vi "数据表比对.vi"(6 "table输入 3":string(combo), 8 "error in (no error)":errorcluster, 9 "查询元素输入":string(combo), 10 "仪器日志参数":string, 11 "table输入":string(combo)) -> (0 "error out":errorcluster, 2 "待发送第一条数据":string[](array[string]), 3 "待发送数据":string[][](table), 4 "获取有效数据":string[][](array[string]))   [LabVIEW 2016]
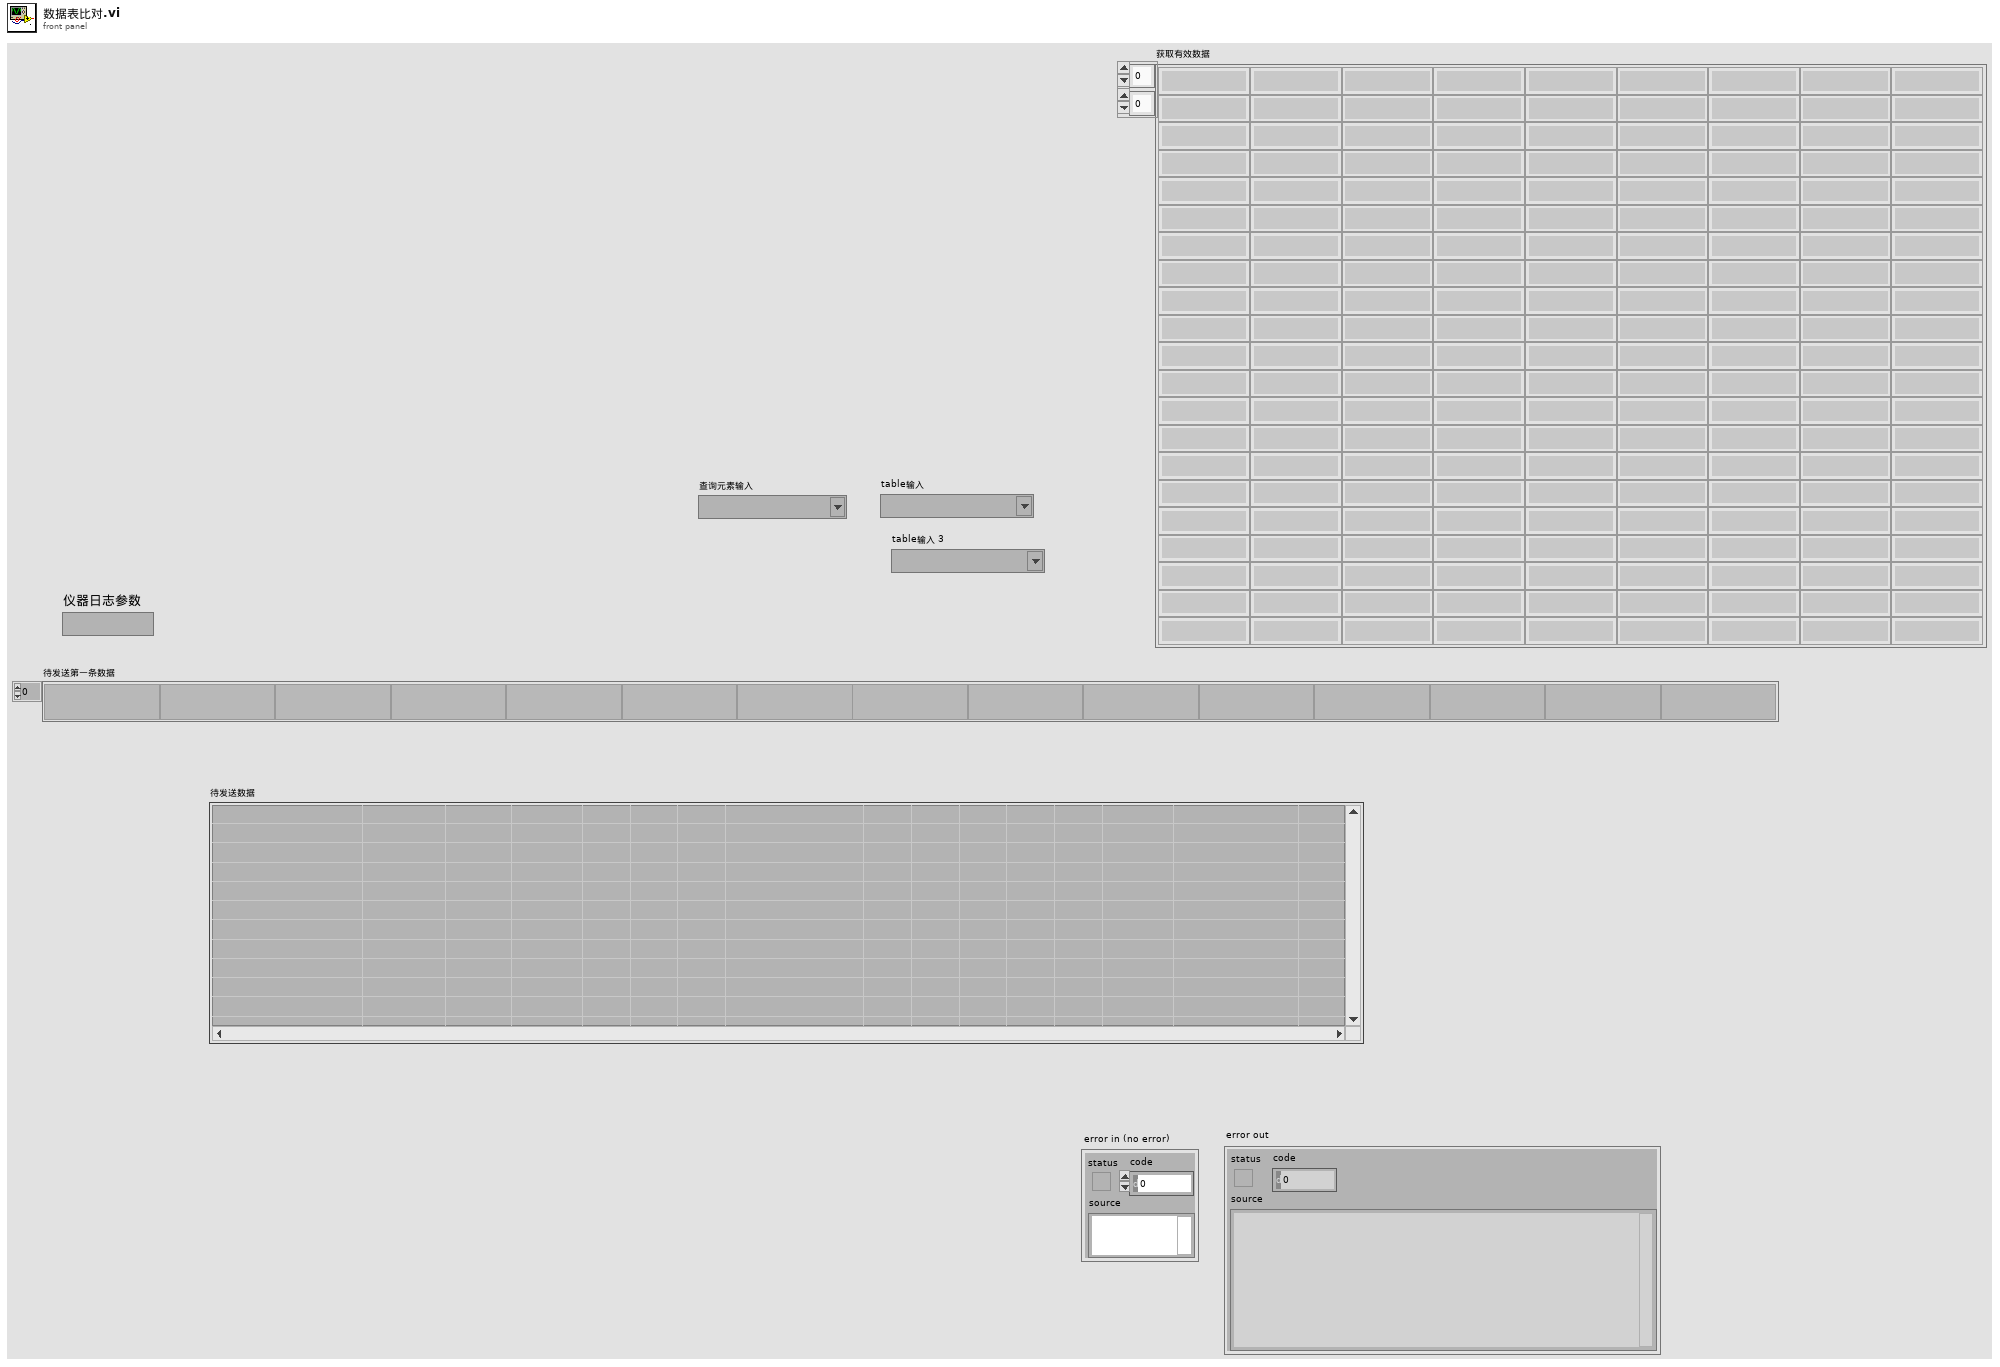
[diagram p1: front panel]
types:
  T1 = typedef "LVDateTimeRec.ctl" = cluster{"秒数的小数部分":dbl, "秒":i32, "分":i32, "时":i32, "日":i32, "月":i32, "年":i32, "天数（周）":i32, "天数（年）":i32, "DST":i32}
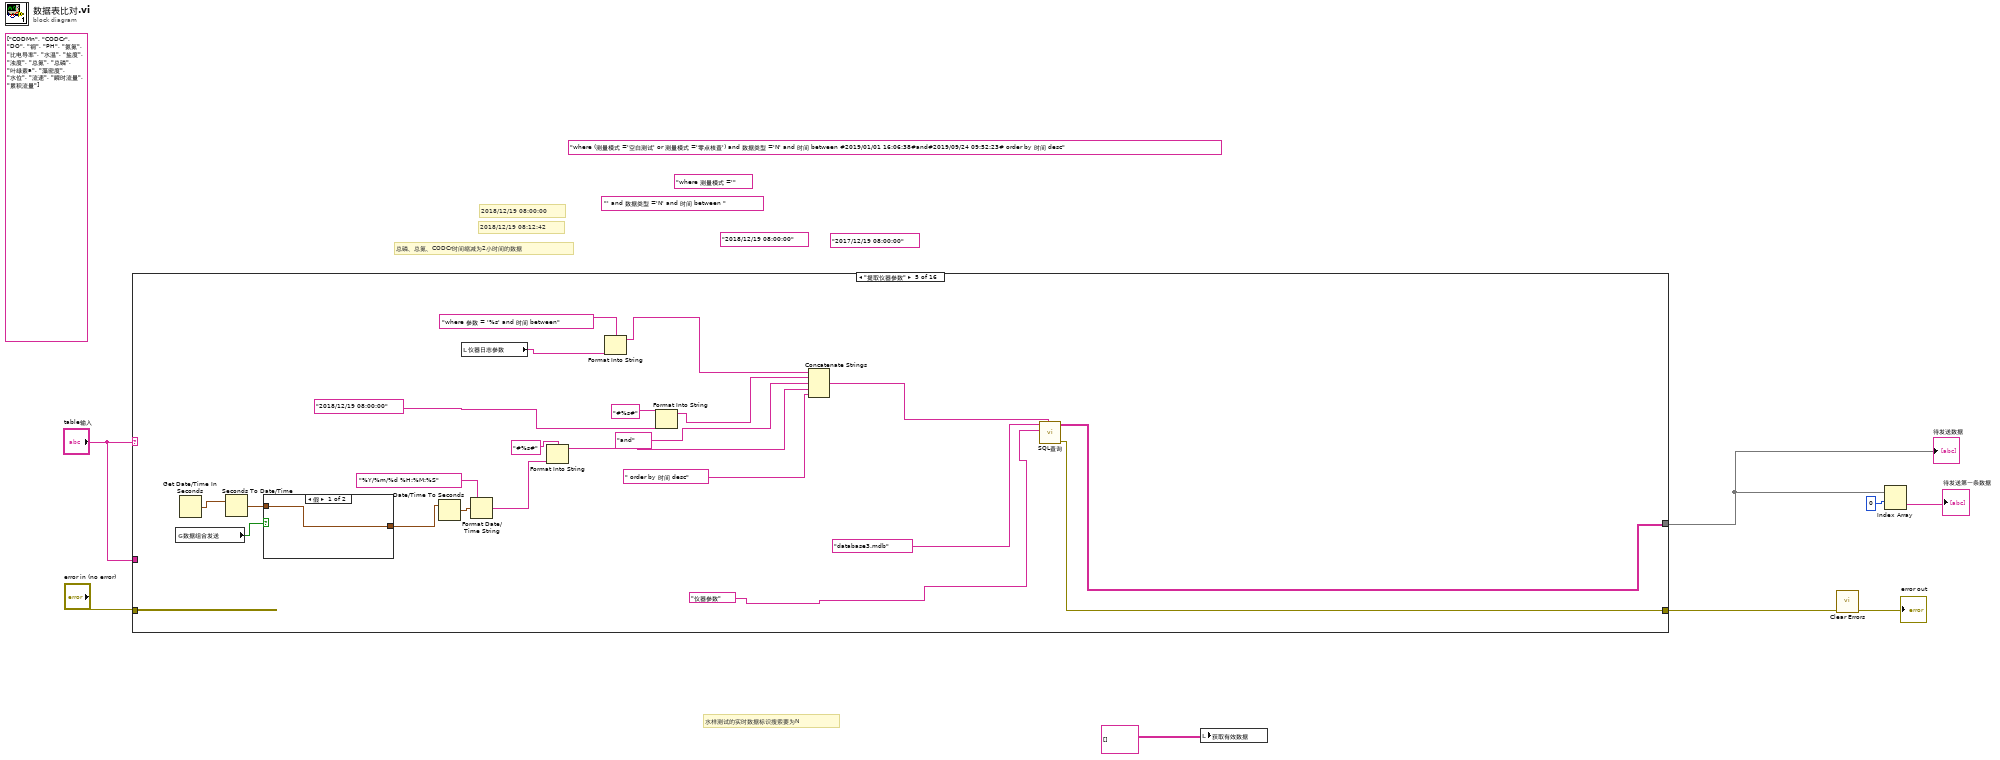
[diagram p0: block diagram]
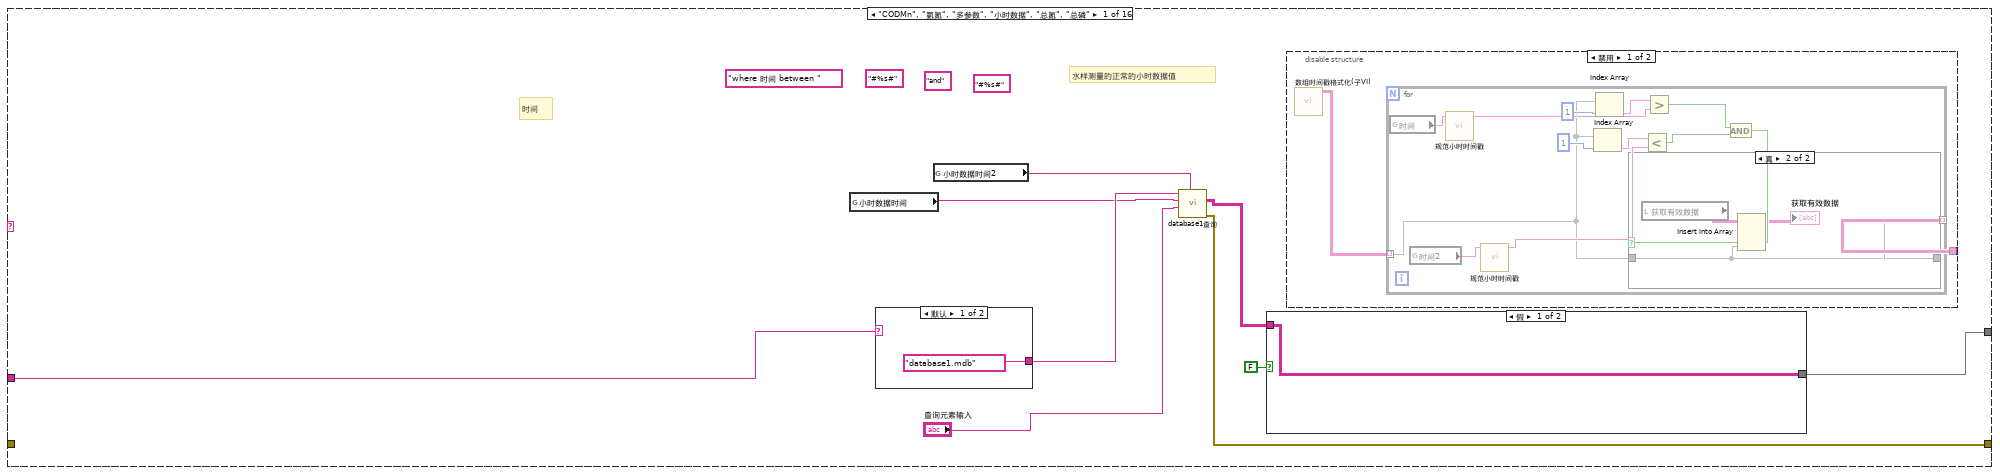
[diagram p2: hidden frame]
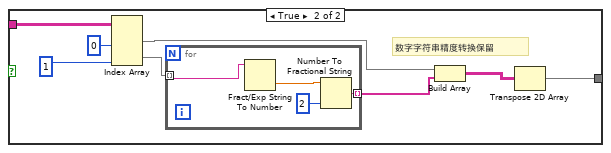
[diagram p3: hidden frame]
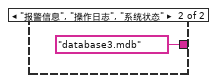
[diagram p6: hidden frame]
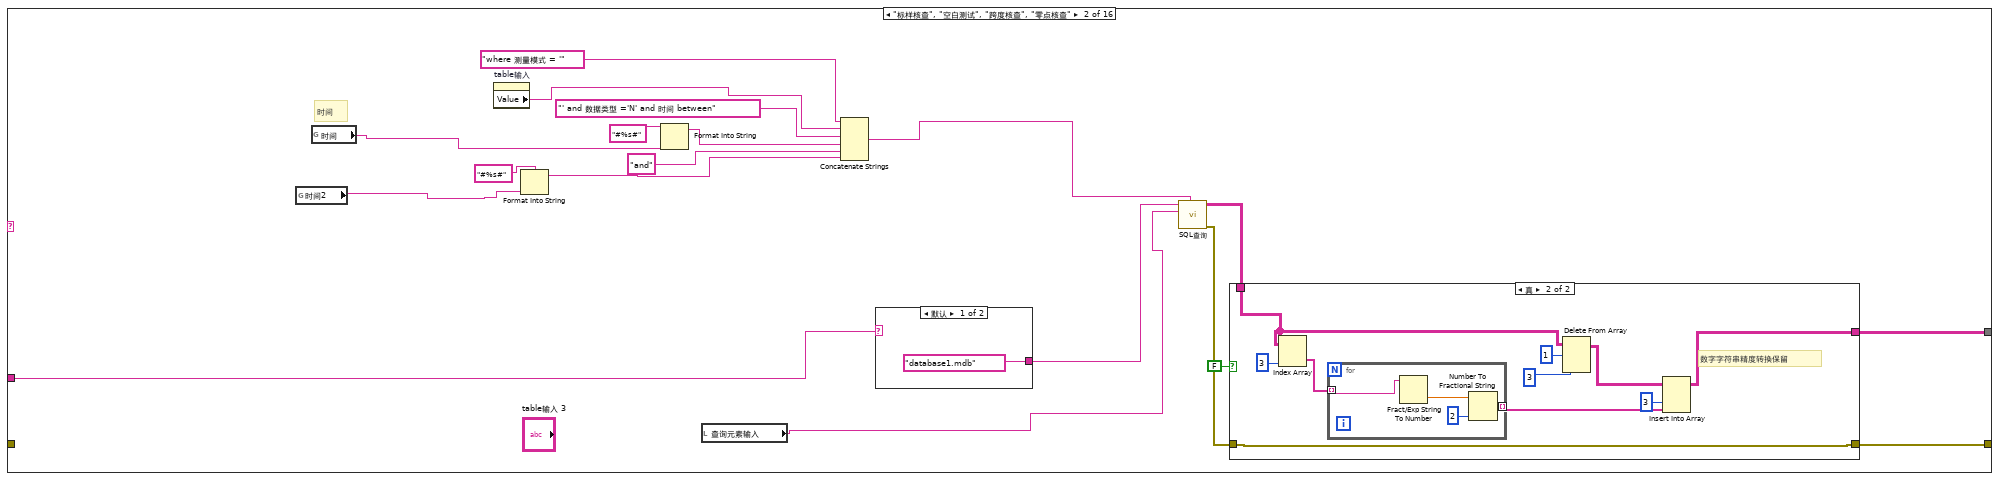
[diagram p7: hidden frame]
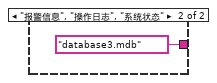
[diagram p9: hidden frame]
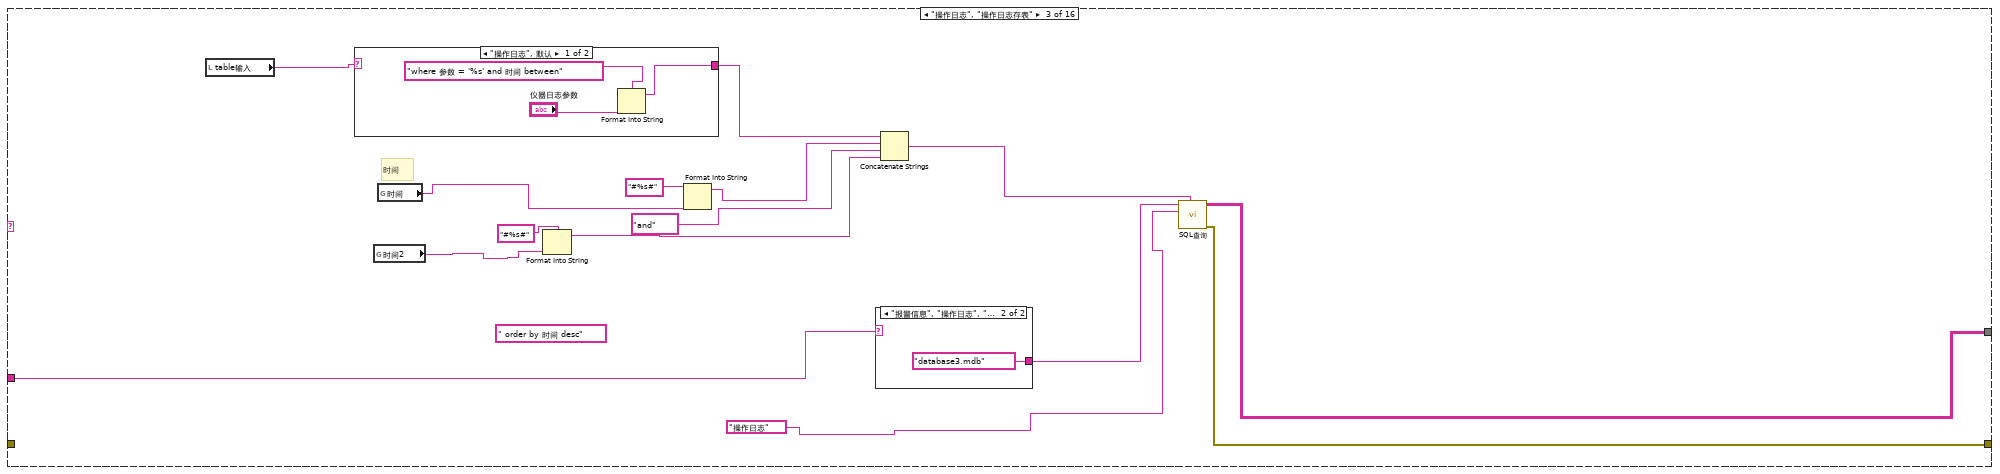
[diagram p10: hidden frame]
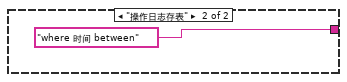
[diagram p11: hidden frame]
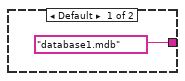
[diagram p12: hidden frame]
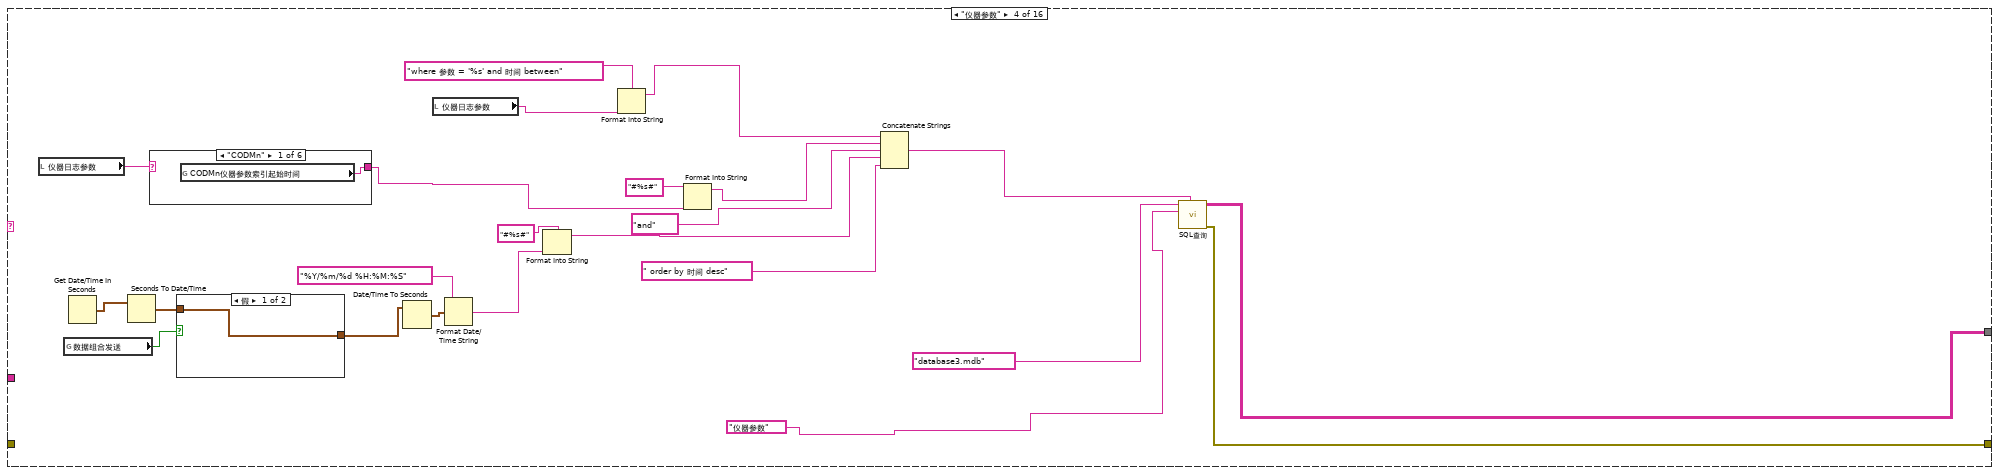
[diagram p13: hidden frame]
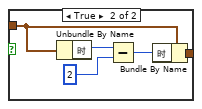
[diagram p14: hidden frame]
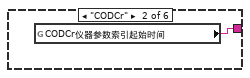
[diagram p15: hidden frame]
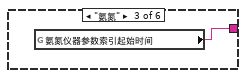
[diagram p16: hidden frame]
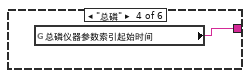
[diagram p17: hidden frame]
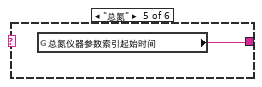
[diagram p18: hidden frame]
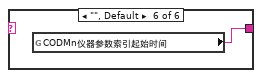
[diagram p19: hidden frame]
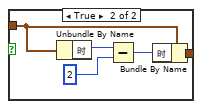
[diagram p20: hidden frame]
diagram:
  (unwired) "' and 数据类型 ='N' and 时间 between "
  (unwired) "where 测量模式 ='" ("condition")
  (unwired) "where (测量模式 ='空白测试' or 测量模式 ='零点核查') and 数据类型 ='N' and 时间 between #2019/01/01 16:06:38#and#2019/09/24 09:52:23# order by 时间 desc" ("condition")
  (unwired) string[] ["CODMn", "CODCr", "DO", "铜", "PH", "氨氮", "比电导率", "水温", "盐度", "浊度", "总氮", "总磷", "叶绿素a", "藻密度", "水位", "流速", "瞬时流量", "累积流量"] ("查询参数数组")
  (unwired) "2017/12/19 08:00:00"
  (unwired) "2018/12/19 08:00:00"
  # "水样测试的实时数据标识搜索要为N"
  # "2018/12/19 08:00:00"
  # "总磷、总氮、CODCr时间缩减为2小时间的数据"
  # "2018/12/19 08:12:42"
  n1 = case shown="\"提取仪器参数\"" "table输入" {
    tunnel: "error in (no error)" -> [_ _ _ _ _ _ _ w232 _ _ _ _ _ _ _ _]
    tunnel: [w14 w55 w100 w130 w164 w186 w219 w232 w247 w343 w390 w444 w499 w542 w585 w625] -> w6
    tunnel: [w10 w58 w98 w128 w162 w184 w217 w230 w250 w346 w393 w447 w502 w545 w588 w627] -> w1
    tunnel: "table输入" -> [w17 w69 w102 _ _ w174 w209 _ _ _ _ _ _ _ _ _]
    frame "CODMn", "氨氮", "多参数", "小时数据", "总氮", "总磷" {
      (unwired) "and" ("字符串")
      (unwired) "#%s#" ("初始字符串")
      (unwired) "#%s#" ("初始字符串")
      (unwired) "where 时间 between " ("condition")
      # "水样测量的正常的小时数据值"
      # "时间"
      n2 = global read "全局 水样时间.vi" "小时数据时间"() -> (w13:string)
      n3 = case shown="默认" w17 {
        tunnel: ["database1.mdb" ("database") "database3.mdb" ("database")] -> w16
        frame Default {
        }
        frame "报警信息", "操作日志", "系统状态" {
        }
      }
      n4 = global read "全局 时间2.vi" "小时数据时间2"() -> (w12:string)
      n5 = call "database1查询.vi"("时间2"=w12, "table"="查询元素输入", "时间1"=w13, "database"=w16) -> ("error out"=w14:errorcluster, "data"=w11:string[][])  [unwired: 4 in, 1 out]
      n6 = case shown="假" FALSE {
        tunnel: w11 -> [w18 w26]
        tunnel: [w18 w19] -> w10
        frame False {
        }
        frame True {
          # "数字字符串精度转换保留"
          n7 = Index Array(array=w26, index (col) #1=0 ("禁用的索引 (列)"), index (col) #2=1 ("索引 (列)")) -> (element #1=w22:string[], element #2=w23:string[])  [unwired: 2 in]
          n8 = for {
            tunnel: w23 -> [w28] mode=indexing
            tunnel: [w27] -> w21 mode=indexing
            n9 = Fract/Exp String To Number(string=w28) -> (number=w29:dbl)  [unwired: 3 in, 1 out]
            n10 = Number To Fractional String(number=w29, precision (6)=i16 2 ("精度(6)")) -> (F-format string=w27:string)  [unwired: 2 in]
          }
          n11 = Build Array(w22, w21) -> (w20:string[][])
          n12 = Transpose 2D Array(2D array=w20) -> (transposed array=w19:string[][])
        }
      }
      n13 = disable-structure shown="禁用" {
        disable-tunnel: [w31 _] -> _
        frame Disabled {
          n14 = call "数组时间戳格式化(子VI).vi"() -> ("待发送数据输出"=w32:string[][])  [unwired: 11 in]
          n15 = for {
            tunnel: w32 -> [w33] mode=indexing
            tunnel: [w35] -> w31 mode=indexing
            n16 = global read "全局 水样时间.vi" "时间"() -> (w39:string)
            n17 = global read "全局 时间2.vi" "时间2"() -> (w37:string)
            n18 = call "规范小时时间戳.vi"("字符串"=w39) -> ("result string"=w38:string)  [unwired: 10 in]
            n19 = call "规范小时时间戳.vi"("字符串"=w37) -> ("result string"=w36:string)  [unwired: 10 in]
            n20 = Index Array(array=w33, index=1 ("索引")) -> (element=w42:string)
            n21 = Index Array(array=w33, index=1 ("索引")) -> (element=w44:string)
            n22 = Less?(x=w42, y=w36) -> (x < y?=w41:bool)
            n23 = Greater?(x=w44, y=w38) -> (0:w40:bool)
            n24 = And(x=w40, y=w41) -> (x .and. y?=w34:bool)
            n25 = case shown="真" w34 {
              tunnel: w33 -> [_ w48]
              tunnel: [_ w48] -> w35
              frame False {
              }
              frame True {
                n26 = local read "获取有效数据"() -> (w47:string[][])
                n27 = Insert Into Array(array=w47, new element=w48) -> (→"获取有效数据":string[][])  [unwired: 2 in]
              }
            }
          }
        }
        frame Enabled {
        }
      }
    }
    frame "标样核查", "空白测试", "跨度核查", "零点核查" {
      # "时间"
      n28 = global read "全局 时间2.vi" "时间2"() -> (w60:string)
      n29 = global read "全局 水样时间.vi" "时间"() -> (w61:string)
      n30 = property on="table输入" class="CmbBox"() -> ("Value"=w51:string)  [unwired: 2 in, 2 out]
      n31 = Format Into String(format string="#%s#" ("初始字符串"), w60) -> (resulting string=w63:string)  [unwired: 2 in, 1 out]
      n32 = Format Into String(format string="#%s#" ("初始字符串"), w61) -> (resulting string=w67:string)  [unwired: 2 in, 1 out]
      n33 = local read "查询元素输入"() -> (w54:string)
      n34 = Concatenate Strings("where 测量模式 = '" ("condition"), w51, "' and 数据类型 ='N' and 时间 between" ("字符串"), w67, "and" ("字符串"), w63) -> (w62:string)
      n35 = case shown="默认" w69 {
        tunnel: ["database1.mdb" ("database") "database3.mdb" ("database")] -> w68
        frame Default {
        }
        frame "报警信息", "操作日志", "系统状态" {
        }
      }
      n36 = call "SQL查询.vi"("condition"=w62, "table输入"=w54, "database"=w68) -> ("error out"=w56:errorcluster, "data"=w59:string[][])  [unwired: 7 in]
      n37 = case shown="真" FALSE {
        tunnel: w59 -> [w71 w74]
        tunnel: [w71 w73] -> w58
        tunnel: [w70 w72] -> w55
        tunnel: w56 -> [w70 w72]
        frame False {
        }
        frame True {
          # "数字字符串精度转换保留"
          n38 = Index Array(array=w74, index (col)=3 ("禁用的索引 (列)")) -> (element=w80:string[])  [unwired: 1 in]
          n39 = for {
            tunnel: w80 -> [w83] mode=indexing
            tunnel: [w82] -> w76 mode=indexing
            n40 = Fract/Exp String To Number(string=w83) -> (number=w84:dbl)  [unwired: 3 in, 1 out]
            n41 = Number To Fractional String(number=w84, precision (6)=i16 2 ("精度(6)")) -> (F-format string=w82:string)  [unwired: 2 in]
          }
          n42 = Delete From Array(array=w74, length=1 ("长度"), index (col)=3 ("禁用的索引 (列)")) -> (array with subset deleted=w77:string[][])  [unwired: 1 in, 1 out]
          n43 = Insert Into Array(array=w77, index (col)=3 ("禁用的索引 (列)"), new element=w76) -> (w73:string[][])  [unwired: 1 in]
        }
      }
    }
    frame "操作日志", "操作日志存表" {
      (unwired) " order by 时间 desc" ("字符串")
      # "时间"
      n44 = local read "table输入"() -> (w90:string)
      n45 = case shown="\"操作日志\", 默认" w90 {
        tunnel: [w103 "where 时间 between" ("condition")] -> w89
        frame "操作日志", Default {
          n46 = Format Into String(format string="where 参数 = '%s' and 时间 between" ("condition"), "仪器日志参数") -> (resulting string=w103:string)  [unwired: 2 in, 1 out]
        }
        frame "操作日志存表" {
        }
      }
      n47 = global read "全局 时间2.vi" "时间2"() -> (w91:string)
      n48 = global read "全局 水样时间.vi" "时间"() -> (w92:string)
      n49 = Format Into String(format string="#%s#" ("初始字符串"), w91) -> (resulting string=w93:string)  [unwired: 2 in, 1 out]
      n50 = Format Into String(format string="#%s#" ("初始字符串"), w92) -> (resulting string=w97:string)  [unwired: 2 in, 1 out]
      n51 = case shown="\"报警信息\", \"操作日志\", \"操作日志存表\", \"系统状态\"" w102 {
        tunnel: ["database1.mdb" ("database") "database3.mdb" ("database")] -> w101
        frame Default {
        }
        frame "报警信息", "操作日志", "操作日志存表", "系统状态" {
        }
      }
      n52 = Concatenate Strings(w89, w97, "and" ("字符串"), w93) -> (w99:string)
      n53 = call "SQL查询.vi"("condition"=w99, "table输入"="操作日志", "database"=w101) -> ("error out"=w100:errorcluster, "data"=w98:string[][])  [unwired: 7 in]
    }
    frame "仪器参数" {
      n54 = local read "仪器日志参数"() -> (w109:string)
      n55 = global read "断电保存全局.vi" "数据组合发送"() -> (w116:bool)
      n56 = Get Date/Time In Seconds() -> (seconds since 1Jan1904=w111:timestamp)
      n57 = Seconds To Date/Time(time stamp (now)=w111) -> (date time rec=w114:T1)  [unwired: 1 in]
      n58 = case shown="\"CODMn\"" w109 {
        tunnel: [w138 w139 w140 w141 w142 w143] -> w117
        frame "CODMn" {
          n59 = global read "全局 时间2.vi" "CODMn仪器参数索引起始时间"() -> (w138:string)
        }
        frame "CODCr" {
          n60 = global read "全局 时间2.vi" "CODCr仪器参数索引起始时间"() -> (w139:string)
        }
        frame "氨氮" {
          n61 = global read "全局 时间2.vi" "氨氮仪器参数索引起始时间"() -> (w140:string)
        }
        frame "总磷" {
          n62 = global read "全局 时间2.vi" "总磷仪器参数索引起始时间"() -> (w141:string)
        }
        frame "总氮" {
          n63 = global read "全局 时间2.vi" "总氮仪器参数索引起始时间"() -> (w142:string)
        }
        frame "", Default {
          n64 = global read "全局 时间2.vi" "CODMn仪器参数索引起始时间"() -> (w143:string)
        }
      }
      n65 = case shown="假" w116 {
        tunnel: w114 -> [w132 w135]
        tunnel: [w132 w133] -> w115
        frame False {
        }
        frame True {
          n66 = Unbundle By Name(w135) -> ("时"=w137:i32)
          n67 = Subtract(x=w137, y=2) -> (x-y=w134:i32)
          n68 = Bundle By Name(cluster=w135, "时"=w134) -> (w133:T1)
        }
      }
      n69 = Date/Time To Seconds(2:w115) -> (0:w112:timestamp)  [unwired: 1 in]
      n70 = local read "仪器日志参数"() -> (w118:string)
      n71 = Format Date/Time String(time format string (%c)="%Y/%m/%d %H:%M:%S" ("时间格式字符串(%c)"), seconds (now)=w112) -> (date/time string=w110:string)  [unwired: 1 in]
      n72 = Format Into String(format string="#%s#" ("初始字符串"), w110) -> (resulting string=w123:string)  [unwired: 2 in, 1 out]
      n73 = Format Into String(format string="where 参数 = '%s' and 时间 between" ("condition"), w118) -> (resulting string=w122:string)  [unwired: 2 in, 1 out]
      n74 = Format Into String(format string="#%s#" ("初始字符串"), w117) -> (resulting string=w127:string)  [unwired: 2 in, 1 out]
      n75 = Concatenate Strings(w122, w127, "and" ("字符串"), w123, " order by 时间 desc" ("字符串")) -> (w129:string)
      n76 = call "SQL查询.vi"("condition"=w129, "table输入"="仪器参数", "database"="database3.mdb") -> ("error out"=w130:errorcluster, "data"=w128:string[][])  [unwired: 7 in]
    }
    frame "提取仪器参数" {
      n77 = global read "断电保存全局.vi" "数据组合发送"() -> (w151:bool)
      n78 = Get Date/Time In Seconds() -> (seconds since 1Jan1904=w146:timestamp)
      n79 = Seconds To Date/Time(time stamp (now)=w146) -> (date time rec=w149:T1)  [unwired: 1 in]
      n80 = case shown="假" w151 {
        tunnel: w149 -> [w166 w169]
        tunnel: [w166 w167] -> w150
        frame False {
        }
        frame True {
          n81 = Unbundle By Name(w169) -> ("时"=w171:i32)
          n82 = Subtract(x=w171, y=2) -> (x-y=w168:i32)
          n83 = Bundle By Name(cluster=w169, "时"=w168) -> (w167:T1)
        }
      }
      n84 = Date/Time To Seconds(2:w150) -> (0:w147:timestamp)  [unwired: 1 in]
      n85 = local read "仪器日志参数"() -> (w152:string)
      n86 = Format Date/Time String(time format string (%c)="%Y/%m/%d %H:%M:%S" ("时间格式字符串(%c)"), seconds (now)=w147) -> (date/time string=w145:string)  [unwired: 1 in]
      n87 = Format Into String(format string="#%s#" ("初始字符串"), w145) -> (resulting string=w157:string)  [unwired: 2 in, 1 out]
      n88 = Format Into String(format string="where 参数 = '%s' and 时间 between" ("condition"), w152) -> (resulting string=w156:string)  [unwired: 2 in, 1 out]
      n89 = Format Into String(format string="#%s#" ("初始字符串"), "2018/12/19 08:00:00") -> (resulting string=w161:string)  [unwired: 2 in, 1 out]
      n90 = Concatenate Strings(w156, w161, "and" ("字符串"), w157, " order by 时间 desc" ("字符串")) -> (w163:string)
      n91 = call "SQL查询.vi"("condition"=w163, "table输入"="仪器参数", "database"="database3.mdb") -> ("error out"=w164:errorcluster, "data"=w162:string[][])  [unwired: 7 in]
    }
    frame "报警信息", "报警信息存表" {
      # "时间"
      n92 = local read "table输入"() -> (w173:string)
      n93 = case shown="\"环境参数\"" w173 {
        tunnel: [w193 w196 "where 时间 between" ("condition")] -> w176
        frame "报警信息", Default {
          n94 = local read "仪器日志参数"() -> (w192:string)
          n95 = Format Into String(format string="where 参数 = '%s' and 时间 between" ("condition"), w192) -> (resulting string=w193:string)  [unwired: 2 in, 1 out]
        }
        frame "环境参数" {
          n96 = local read "仪器日志参数"() -> (w195:string)
          n97 = Format Into String(format string="where 参数 = '%s' and 时间 between" ("condition"), w195) -> (resulting string=w196:string)  [unwired: 2 in, 1 out]
        }
        frame "报警信息存表" {
        }
      }
      n98 = global read "全局 时间2.vi" "时间2"() -> (w177:string)
      n99 = global read "全局 水样时间.vi" "时间"() -> (w178:string)
      n100 = case shown="\"环境参数\"" w173 {
        tunnel: [" order by 时间 desc" ("字符串") "" ("仪器日志参数")] -> w172
        frame "环境参数" {
        }
        frame "报警信息", Default {
        }
      }
      n101 = Format Into String(format string="#%s#" ("初始字符串"), w177) -> (resulting string=w179:string)  [unwired: 2 in, 1 out]
      n102 = case shown="\"报警信息\", 默认" w174 {
        tunnel: [w190 "报警信息" ("table输入")] -> w175
        frame "环境参数" {
          n103 = local read "仪器日志参数"() -> (w190:string)
        }
        frame "报警信息", Default {
        }
      }
      n104 = Format Into String(format string="#%s#" ("初始字符串"), w178) -> (resulting string=w183:string)  [unwired: 2 in, 1 out]
      n105 = case shown="默认" w174 {
        tunnel: ["database1.mdb" ("database") "database3.mdb" ("database")] -> w187
        frame Default {
        }
        frame "报警信息", "报警信息存表", "操作日志", "系统状态" {
        }
      }
      n106 = Concatenate Strings(w176, w183, "and" ("字符串"), w179, w172) -> (w185:string)
      n107 = call "SQL查询.vi"("condition"=w185, "table输入"=w175, "database"=w187) -> ("error out"=w186:errorcluster, "data"=w184:string[][])  [unwired: 7 in]
    }
    frame "环境参数" {
      n108 = local read "table输入"() -> (w208:string)
      n109 = Get Date/Time In Seconds() -> (seconds since 1Jan1904=w205:timestamp)
      n110 = Seconds To Date/Time(time stamp (now)=w205) -> (date time rec=w202:T1)  [unwired: 1 in]
      n111 = case shown="\"环境参数\"" w208 {
        tunnel: [w224 "where 时间 between" ("condition") "where 时间 between" ("condition")] -> w211
        frame "报警信息", Default {
          n112 = local read "仪器日志参数"() -> (w223:string)
          n113 = Format Into String(format string="where 参数 = '%s' and 时间 between" ("condition"), w223) -> (resulting string=w224:string)  [unwired: 2 in, 1 out]
        }
        frame "环境参数" {
        }
        frame "报警信息存表" {
        }
      }
      n114 = Date/Time To Seconds(2:w202) -> (0:w204:timestamp)  [unwired: 1 in]
      n115 = Format Date/Time String(time format string (%c)="%Y/%m/%d %H:%M:%S" ("时间格式字符串(%c)"), seconds (now)=w204) -> (date/time string=w201:string)  [unwired: 1 in]
      n116 = Format Into String(format string="#%s#" ("初始字符串"), w201) -> (resulting string=w212:string)  [unwired: 2 in, 1 out]
      n117 = case shown="\"环境参数\"" w209 {
        tunnel: [w221 "报警信息" ("table输入")] -> w210
        frame "环境参数" {
          n118 = local read "仪器日志参数"() -> (w221:string)
        }
        frame "报警信息", Default {
        }
      }
      n119 = Format Into String(format string="#%s#" ("初始字符串"), "1904/01/01 00:00:00") -> (resulting string=w216:string)  [unwired: 2 in, 1 out]
      n120 = case shown="默认" w209 {
        tunnel: ["database1.mdb" ("database") "database3.mdb" ("database")] -> w220
        frame Default {
        }
        frame "报警信息", "报警信息存表", "操作日志", "系统状态" {
        }
      }
      n121 = Concatenate Strings(w211, w216, "and" ("字符串"), w212, " order by 时间 desc" ("字符串")) -> (w218:string)
      n122 = call "SQL查询.vi"("condition"=w218, "table输入"=w210, "database"=w220) -> ("error out"=w219:errorcluster, "data"=w217:string[][])  [unwired: 7 in]
    }
    frame Default {
      # "时间格式转换"
      n123 = local read "待发送数据"() -> (w231:string[][])
      n124 = call "数组时间戳格式化(子VI).vi"("待发送数据输入"=w231) -> ("待发送数据输出"=w230:string[][])  [unwired: 10 in]
    }
    frame "实时数据" {
      # "空白测试or零点核查要加括号"
      # "上传本地时间点的实时数据"
      # "上传质控数据（空白测试，跨度核查，核查数据，平行样数据）"
      n125 = global read "全局 实时数据参数.vi" "实时数据参数"() -> (w242:string)
      n126 = global read "断电保存全局.vi" "数据组合发送"() -> (w234:bool)
      n127 = Get Date/Time In Seconds() -> (seconds since 1Jan1904=w241:timestamp)
      n128 = case shown="\"空白测试\"" w242 {
        tunnel: [w267 w289 w300 w306] -> w243
        tunnel: w242 -> [w263 w287 _ w302]
        tunnel: [w266 w283 w296 w301] -> w237
        frame "水样测试" {
          n129 = Get Date/Time In Seconds() -> (seconds since 1Jan1904=w275:timestamp)
          n130 = local read "查询元素输入"() -> (w268:string)
          n131 = Format Date/Time String(time format string (%c)="%Y%m%d%H%M%S%3u" ("时间格式字符串(%c)"), seconds (now)=w275) -> (date/time string=w273:string)  [unwired: 1 in]
          n132 = Replace Substring(2:8 ("长度（子字符串长度）"), 3:10 ("偏移量(0)"), 4:"0000" ("子字符串(\"\")"), 5:w273) -> (1:w269:string)  [unwired: 1 out]
          n133 = case shown="默认" w268 {
            tunnel: w269 -> [w277 w280 _]
            tunnel: [w276 w281 w282] -> w267
            frame Default {
              n134 = Search and Replace String(input string=w277, search string="." ("搜索字符串")) -> (result string=w278:string)  [unwired: 6 in, 3 out]
              n135 = call "格式时间字符串.vi"("字符串"=w278) -> ("连接的字符串"=w276:string)  [unwired: 10 in]
            }
            frame "CODCr", "CODMn", "累积流量", "总氮", "总磷" {
              n136 = call "实时数据查询用2小时间的数据.vi"("字符串"=w280) -> ("连接的字符串"=w281:string)  [unwired: 10 in]
            }
            frame "CODCr加标回收率", "CODMn加标回收率", "氨氮加标回收率", "总氮加标回收率", "总磷加标回收率" {
              n137 = global read "全局 时间2.vi" "加标回收索引起始时间"() -> (w282:string)
            }
          }
          n138 = Concatenate Strings("where 测量模式 ='" ("condition"), w263, "' and 数据类型 ='N' and 时间 between ") -> (w266:string)
        }
        frame "空白测试" {
          n139 = local read "查询元素输入"() -> (w288:string)
          n140 = case shown="\"氨氮\"" w288 {
            tunnel: [w290 w291 w292 w293 w294 w295] -> w289
            frame "CODMn" {
              n141 = global read "全局 时间2.vi" "CODMn零点核查索引起始时间"() -> (w290:string)
            }
            frame "CODCr" {
              n142 = global read "全局 时间2.vi" "CODCr零点核查索引起始时间"() -> (w291:string)
            }
            frame "氨氮" {
              n143 = global read "全局 时间2.vi" "氨氮零点核查索引起始时间"() -> (w292:string)
            }
            frame "总磷" {
              n144 = global read "全局 时间2.vi" "总磷零点核查索引起始时间"() -> (w293:string)
            }
            frame "总氮" {
              n145 = global read "全局 时间2.vi" "总氮零点核查索引起始时间"() -> (w294:string)
            }
            frame "", Default {
              n146 = global read "全局 时间2.vi" "零点核查索引起始时间"() -> (w295:string)
            }
          }
          n147 = Concatenate Strings("where (测量模式 ='" ("condition"), w287, "' or 测量模式 = '零点核查", "') and 数据类型 ='N' and 时间 between ") -> (w283:string)
        }
        frame "核查数据" {
          n148 = global read "全局 时间2.vi" "标样核查索引起始时间"() -> (w300:string)
          n149 = Concatenate Strings("where 测量模式 ='" ("condition"), "标样核查" ("实时数据参数"), "' and 数据类型 ='N' and 时间 between ") -> (w296:string)
        }
        frame "跨度核查", Default {
          n150 = local read "查询元素输入"() -> (w305:string)
          n151 = case shown="\"氨氮\"" w305 {
            tunnel: [w307 w308 w309 w310 w311 w312] -> w306
            frame "CODMn" {
              n152 = global read "全局 时间2.vi" "CODMn跨度核查索引起始时间"() -> (w307:string)
            }
            frame "CODCr" {
              n153 = global read "全局 时间2.vi" "CODCr跨度核查索引起始时间"() -> (w308:string)
            }
            frame "氨氮" {
              n154 = global read "全局 时间2.vi" "氨氮跨度核查索引起始时间"() -> (w309:string)
            }
            frame "总磷" {
              n155 = global read "全局 时间2.vi" "总磷跨度核查索引起始时间"() -> (w310:string)
            }
            frame "总氮" {
              n156 = global read "全局 时间2.vi" "总氮跨度核查索引起始时间"() -> (w311:string)
            }
            frame "", Default {
              n157 = global read "全局 时间2.vi" "跨度核查索引起始时间"() -> (w312:string)
            }
          }
          n158 = Concatenate Strings("where 测量模式 ='" ("condition"), w302, "' and 数据类型 ='N' and 时间 between ") -> (w301:string)
        }
      }
      n159 = Seconds To Date/Time(time stamp (now)=w241) -> (date time rec=w236:T1)  [unwired: 1 in]
      n160 = case shown="假" w234 {
        tunnel: w236 -> [w257 w260]
        tunnel: [w257 w258] -> w235
        frame False {
        }
        frame True {
          n161 = Unbundle By Name(w260) -> ("时"=w262:i32)
          n162 = Subtract(x=w262, y=2) -> (x-y=w259:i32)
          n163 = Bundle By Name(cluster=w260, "时"=w259) -> (w258:T1)
        }
      }
      n164 = Date/Time To Seconds(2:w235) -> (0:w240:timestamp)  [unwired: 1 in]
      n165 = Format Date/Time String(time format string (%c)="%Y/%m/%d %H:%M:%S" ("时间格式字符串(%c)"), seconds (now)=w240) -> (date/time string=w238:string)  [unwired: 1 in]
      n166 = local read "查询元素输入"() -> (w246:string)
      n167 = Format Into String(format string="#%s#" ("初始字符串"), w238) -> (resulting string=w252:string)  [unwired: 2 in, 1 out]
      n168 = Format Into String(format string="#%s#" ("初始字符串"), w243) -> (resulting string=w256:string)  [unwired: 2 in, 1 out]
      n169 = Concatenate Strings(w237, w256, "and" ("字符串"), w252, " order by 时间 desc" ("字符串")) -> (w245:string)
      n170 = call "SQL查询.vi"("condition"=w245, "table输入"=w246, "database"="database1.mdb") -> ("error out"=w248:errorcluster, "data"=w244:string[][])  [unwired: 7 in]
      n171 = case shown="假" FALSE {
        tunnel: [w317 w320] -> w250
        tunnel: w244 -> [w317 w319]
        tunnel: w248 -> [w316 w318]
        tunnel: [w316 w318] -> w247
        frame False {
        }
        frame True {
          # "数字字符串精度转换保留"
          n172 = Index Array(array=w319, index (col)=3 ("禁用的索引 (列)")) -> (element=w326:string[])  [unwired: 1 in]
          n173 = for {
            tunnel: w326 -> [w329] mode=indexing
            tunnel: [w328] -> w322 mode=indexing
            n174 = Fract/Exp String To Number(string=w329) -> (number=w330:dbl)  [unwired: 3 in, 1 out]
            n175 = Number To Fractional String(number=w330, precision (6)=i16 2 ("精度(6)")) -> (F-format string=w328:string)  [unwired: 2 in]
          }
          n176 = Delete From Array(array=w319, length=1 ("长度"), index (col)=3 ("禁用的索引 (列)")) -> (array with subset deleted=w323:string[][])  [unwired: 1 in, 1 out]
          n177 = Insert Into Array(array=w323, index (col)=3 ("禁用的索引 (列)"), new element=w322) -> (w320:string[][])  [unwired: 1 in]
        }
      }
      n178 = case shown="默认" w246 {
        tunnel: w246 -> [_ w315]
        tunnel: w245 -> [_ w314]
        tunnel: w244 -> [_ w313]
        frame Default {
        }
        frame "CODCr", "总氮", "总磷" {
          n179 = global write "全局 实时数据参数.vi" "参数"(w315) -> ()
          n180 = global write "全局 实时数据参数.vi" "连接的字符串"(w314) -> ()
          n181 = global write "全局 实时数据参数.vi" "data"(w313) -> ()
        }
      }
    }
    frame "加标回收" {
      w338 = "加标回收率" ("字符串")
      # "上传本地时间点的实时数据"
      # "上传加标回收数据"
      n182 = global read "全局 数据发送重叠.vi" "掉线指示灯"() -> (w339:bool)
      n183 = case shown="假" w339 {
        tunnel: [w355 w359] -> w340
        frame False {
          n184 = global read "全局 数据发送重叠.vi" "数据发送重叠"() -> (w356:bool)
          n185 = case shown="假" w356 {
            tunnel: [w357 w358] -> w355
            frame False {
              n186 = global read "全局 时间2.vi" "加标回收索引起始时间"() -> (w357:string)
            }
            frame True {
              n187 = global read "全局 数据发送重叠.vi" "数据发送重叠开始时间戳"() -> (w358:string)
            }
          }
        }
        frame True {
          n188 = global read "全局 数据发送重叠.vi" "TCP掉线时间节点"() -> (w359:string)
        }
      }
      n189 = Get Date/Time In Seconds() -> (seconds since 1Jan1904=w336:timestamp)
      n190 = Seconds To Date/Time(time stamp (now)=w336) -> (date time rec=w333:T1)  [unwired: 1 in]
      n191 = Date/Time To Seconds(2:w333) -> (0:w335:timestamp)  [unwired: 1 in]
      n192 = Format Date/Time String(time format string (%c)="%Y/%m/%d %H:%M:%S" ("时间格式字符串(%c)"), seconds (now)=w335) -> (date/time string=w332:string)  [unwired: 1 in]
      n193 = local read "查询元素输入"() -> (w337:string)
      n194 = Format Into String(format string="#%s#" ("初始字符串"), w332) -> (resulting string=w350:string)  [unwired: 2 in, 1 out]
      n195 = Format Into String(format string="#%s#" ("初始字符串"), w340) -> (resulting string=w354:string)  [unwired: 2 in, 1 out]
      n196 = Concatenate Strings("where 参数 ='" ("condition"), w337, "' and 时间 between ", w354, "and" ("字符串"), w350) -> (w342:string)
      n197 = call "SQL查询.vi"("condition"=w342, "table输入"=w338, "database"="database1.mdb") -> ("error out"=w344:errorcluster, "data"=w341:string[][])  [unwired: 7 in]
      n198 = case shown="假" FALSE {
        tunnel: [w364 w367] -> w346
        tunnel: w341 -> [w364 w366]
        tunnel: w344 -> [w363 w365]
        tunnel: [w363 w365] -> w343
        frame False {
        }
        frame True {
          # "数字字符串精度转换保留"
          n199 = Index Array(array=w366, index (col)=3 ("禁用的索引 (列)")) -> (element=w373:string[])  [unwired: 1 in]
          n200 = for {
            tunnel: w373 -> [w376] mode=indexing
            tunnel: [w375] -> w369 mode=indexing
            n201 = Fract/Exp String To Number(string=w376) -> (number=w377:dbl)  [unwired: 3 in, 1 out]
            n202 = Number To Fractional String(number=w377, precision (6)=i16 2 ("精度(6)")) -> (F-format string=w375:string)  [unwired: 2 in]
          }
          n203 = Delete From Array(array=w366, length=1 ("长度"), index (col)=3 ("禁用的索引 (列)")) -> (array with subset deleted=w370:string[][])  [unwired: 1 in, 1 out]
          n204 = Insert Into Array(array=w370, index (col)=3 ("禁用的索引 (列)"), new element=w369) -> (w367:string[][])  [unwired: 1 in]
        }
      }
      n205 = case shown="\"CODCr\", \"总氮\", \"总磷\"" w338 {
        tunnel: w338 -> [_ w362]
        tunnel: w342 -> [_ w361]
        tunnel: w341 -> [_ w360]
        frame Default {
        }
        frame "CODCr", "总氮", "总磷" {
          n206 = global write "全局 实时数据参数.vi" "参数"(w362) -> ()
          n207 = global write "全局 实时数据参数.vi" "连接的字符串"(w361) -> ()
          n208 = global write "全局 实时数据参数.vi" "data"(w360) -> ()
        }
      }
    }
    frame "平行样测试" {
      w385 = "平行样测试" ("字符串")
      # "上传本地时间点的实时数据"
      # "上传平行样数据"
      n209 = global read "全局 数据发送重叠.vi" "掉线指示灯"() -> (w386:bool)
      n210 = case shown="假" w386 {
        tunnel: [w402 w413] -> w387
        frame False {
          n211 = global read "全局 数据发送重叠.vi" "数据发送重叠"() -> (w403:bool)
          n212 = case shown="假" w403 {
            tunnel: [w404 w412] -> w402
            frame False {
              n213 = local read "查询元素输入"() -> (w405:string)
              n214 = case shown="\"CODCr\"" w405 {
                tunnel: [w406 w407 w408 w409 w410 w411] -> w404
                frame "CODMn" {
                  n215 = global read "全局 时间2.vi" "CODMn平行样索引起始时间"() -> (w406:string)
                }
                frame "CODCr" {
                  n216 = global read "全局 时间2.vi" "CODCr平行样索引起始时间"() -> (w407:string)
                }
                frame "氨氮" {
                  n217 = global read "全局 时间2.vi" "氨氮平行样索引起始时间"() -> (w408:string)
                }
                frame "总磷" {
                  n218 = global read "全局 时间2.vi" "总磷平行样索引起始时间"() -> (w409:string)
                }
                frame "总氮" {
                  n219 = global read "全局 时间2.vi" "总磷平行样索引起始时间"() -> (w410:string)
                }
                frame "", Default {
                  n220 = global read "全局 时间2.vi" "平行样索引起始时间"() -> (w411:string)
                }
              }
            }
            frame True {
              n221 = global read "全局 数据发送重叠.vi" "数据发送重叠开始时间戳"() -> (w412:string)
            }
          }
        }
        frame True {
          n222 = global read "全局 数据发送重叠.vi" "TCP掉线时间节点"() -> (w413:string)
        }
      }
      n223 = Get Date/Time In Seconds() -> (seconds since 1Jan1904=w383:timestamp)
      n224 = Seconds To Date/Time(time stamp (now)=w383) -> (date time rec=w380:T1)  [unwired: 1 in]
      n225 = Date/Time To Seconds(2:w380) -> (0:w382:timestamp)  [unwired: 1 in]
      n226 = Format Date/Time String(time format string (%c)="%Y/%m/%d %H:%M:%S" ("时间格式字符串(%c)"), seconds (now)=w382) -> (date/time string=w379:string)  [unwired: 1 in]
      n227 = local read "查询元素输入"() -> (w384:string)
      n228 = Format Into String(format string="#%s#" ("初始字符串"), w379) -> (resulting string=w397:string)  [unwired: 2 in, 1 out]
      n229 = Format Into String(format string="#%s#" ("初始字符串"), w387) -> (resulting string=w401:string)  [unwired: 2 in, 1 out]
      n230 = Concatenate Strings("where 参数 ='" ("condition"), w384, "' and 时间 between ", w401, "and" ("字符串"), w397) -> (w389:string)
      n231 = call "SQL查询.vi"("condition"=w389, "table输入"=w385, "database"="database1.mdb") -> ("error out"=w391:errorcluster, "data"=w388:string[][])  [unwired: 7 in]
      n232 = case shown="假" FALSE {
        tunnel: [w418 w421] -> w393
        tunnel: w388 -> [w418 w420]
        tunnel: w391 -> [w417 w419]
        tunnel: [w417 w419] -> w390
        frame False {
        }
        frame True {
          # "数字字符串精度转换保留"
          n233 = Index Array(array=w420, index (col)=3 ("禁用的索引 (列)")) -> (element=w427:string[])  [unwired: 1 in]
          n234 = for {
            tunnel: w427 -> [w430] mode=indexing
            tunnel: [w429] -> w423 mode=indexing
            n235 = Fract/Exp String To Number(string=w430) -> (number=w431:dbl)  [unwired: 3 in, 1 out]
            n236 = Number To Fractional String(number=w431, precision (6)=i16 2 ("精度(6)")) -> (F-format string=w429:string)  [unwired: 2 in]
          }
          n237 = Delete From Array(array=w420, length=1 ("长度"), index (col)=3 ("禁用的索引 (列)")) -> (array with subset deleted=w424:string[][])  [unwired: 1 in, 1 out]
          n238 = Insert Into Array(array=w424, index (col)=3 ("禁用的索引 (列)"), new element=w423) -> (w421:string[][])  [unwired: 1 in]
        }
      }
      n239 = case shown="默认" w385 {
        tunnel: w385 -> [_ w416]
        tunnel: w389 -> [_ w415]
        tunnel: w388 -> [_ w414]
        frame Default {
        }
        frame "CODCr", "总氮", "总磷" {
          n240 = global write "全局 实时数据参数.vi" "参数"(w416) -> ()
          n241 = global write "全局 实时数据参数.vi" "连接的字符串"(w415) -> ()
          n242 = global write "全局 实时数据参数.vi" "data"(w414) -> ()
        }
      }
    }
    frame "集成干预测试" {
      w439 = "集成干预测试" ("字符串")
      # "上传本地时间点的实时数据"
      # "上传集成干预数据"
      n243 = global read "全局 数据发送重叠.vi" "掉线指示灯"() -> (w440:bool)
      n244 = case shown="假" w440 {
        tunnel: [w456 w472] -> w441
        frame False {
          n245 = global read "全局 数据发送重叠.vi" "数据发送重叠"() -> (w457:bool)
          n246 = case shown="假" w457 {
            tunnel: [w458 w471] -> w456
            frame False {
              n247 = local read "查询元素输入"() -> (w459:string)
              n248 = case shown="\"浊度\"" w459 {
                tunnel: [w460 w461 w462 w463 w464 w465 w466 w467 w468 w469 w470] -> w458
                frame "CODMn" {
                  n249 = global read "全局 时间2.vi" "CODMn集成干预索引起始时间"() -> (w460:string)
                }
                frame "CODCr" {
                  n250 = global read "全局 时间2.vi" "CODCr集成干预索引起始时间"() -> (w461:string)
                }
                frame "氨氮" {
                  n251 = global read "全局 时间2.vi" "氨氮集成干预索引起始时间"() -> (w462:string)
                }
                frame "总磷" {
                  n252 = global read "全局 时间2.vi" "总磷集成干预索引起始时间"() -> (w463:string)
                }
                frame "总氮" {
                  n253 = global read "全局 时间2.vi" "总氮集成干预索引起始时间"() -> (w464:string)
                }
                frame "DO" {
                  n254 = global read "全局 时间2.vi" "DO集成干预索引起始时间"() -> (w465:string)
                }
                frame "PH" {
                  n255 = global read "全局 时间2.vi" "PH集成干预索引起始时间"() -> (w466:string)
                }
                frame "比电导率" {
                  n256 = global read "全局 时间2.vi" "比电导率集成干预索引起始时间"() -> (w467:string)
                }
                frame "水温" {
                  n257 = global read "全局 时间2.vi" "水温集成干预索引起始时间"() -> (w468:string)
                }
                frame "浊度" {
                  n258 = global read "全局 时间2.vi" "浊度集成干预索引起始时间"() -> (w469:string)
                }
                frame "", Default {
                  n259 = global read "全局 时间2.vi" "平行样索引起始时间"() -> (w470:string)
                }
              }
            }
            frame True {
              n260 = global read "全局 数据发送重叠.vi" "数据发送重叠开始时间戳"() -> (w471:string)
            }
          }
        }
        frame True {
          n261 = global read "全局 数据发送重叠.vi" "TCP掉线时间节点"() -> (w472:string)
        }
      }
      n262 = Get Date/Time In Seconds() -> (seconds since 1Jan1904=w437:timestamp)
      n263 = Seconds To Date/Time(time stamp (now)=w437) -> (date time rec=w434:T1)  [unwired: 1 in]
      n264 = Date/Time To Seconds(2:w434) -> (0:w436:timestamp)  [unwired: 1 in]
      n265 = Format Date/Time String(time format string (%c)="%Y/%m/%d %H:%M:%S" ("时间格式字符串(%c)"), seconds (now)=w436) -> (date/time string=w433:string)  [unwired: 1 in]
      n266 = local read "查询元素输入"() -> (w438:string)
      n267 = Format Into String(format string="#%s#" ("初始字符串"), w433) -> (resulting string=w451:string)  [unwired: 2 in, 1 out]
      n268 = Format Into String(format string="#%s#" ("初始字符串"), w441) -> (resulting string=w455:string)  [unwired: 2 in, 1 out]
      n269 = Concatenate Strings("where 参数 ='" ("condition"), w438, "' and 时间 between ", w455, "and" ("字符串"), w451) -> (w443:string)
      n270 = call "SQL查询.vi"("condition"=w443, "table输入"=w439, "database"="database1.mdb") -> ("error out"=w445:errorcluster, "data"=w442:string[][])  [unwired: 7 in]
      n271 = case shown="假" FALSE {
        tunnel: [w477 w480] -> w447
        tunnel: w442 -> [w477 w479]
        tunnel: w445 -> [w476 w478]
        tunnel: [w476 w478] -> w444
        frame False {
        }
        frame True {
          # "数字字符串精度转换保留"
          n272 = Index Array(array=w479, index (col)=3 ("禁用的索引 (列)")) -> (element=w486:string[])  [unwired: 1 in]
          n273 = for {
            tunnel: w486 -> [w489] mode=indexing
            tunnel: [w488] -> w482 mode=indexing
            n274 = Fract/Exp String To Number(string=w489) -> (number=w490:dbl)  [unwired: 3 in, 1 out]
            n275 = Number To Fractional String(number=w490, precision (6)=i16 2 ("精度(6)")) -> (F-format string=w488:string)  [unwired: 2 in]
          }
          n276 = Delete From Array(array=w479, length=1 ("长度"), index (col)=3 ("禁用的索引 (列)")) -> (array with subset deleted=w483:string[][])  [unwired: 1 in, 1 out]
          n277 = Insert Into Array(array=w483, index (col)=3 ("禁用的索引 (列)"), new element=w482) -> (w480:string[][])  [unwired: 1 in]
        }
      }
      n278 = case shown="默认" w439 {
        tunnel: w439 -> [_ w475]
        tunnel: w443 -> [_ w474]
        tunnel: w442 -> [_ w473]
        frame Default {
        }
        frame "CODCr", "总氮", "总磷" {
          n279 = global write "全局 实时数据参数.vi" "参数"(w475) -> ()
          n280 = global write "全局 实时数据参数.vi" "连接的字符串"(w474) -> ()
          n281 = global write "全局 实时数据参数.vi" "data"(w473) -> ()
        }
      }
    }
    frame "提取加标回收" {
      w494 = "加标回收率" ("字符串")
      # "上传本地时间点的实时数据"
      n282 = global read "全局 数据发送重叠.vi" "掉线指示灯"() -> (w495:bool)
      n283 = case shown="假" w495 {
        tunnel: [w511 w515] -> w496
        frame False {
          n284 = global read "全局 数据发送重叠.vi" "数据发送重叠"() -> (w512:bool)
          n285 = case shown="假" w512 {
            tunnel: [w513 w514] -> w511
            frame False {
              n286 = global read "起始时间.vi" "起始时间"() -> (w513:string)
            }
            frame True {
              n287 = global read "全局 数据发送重叠.vi" "数据发送重叠开始时间戳"() -> (w514:string)
            }
          }
        }
        frame True {
          n288 = global read "全局 数据发送重叠.vi" "TCP掉线时间节点"() -> (w515:string)
        }
      }
      n289 = global read "起始时间.vi" "结束时间"() -> (w492:string)
      n290 = local read "查询元素输入"() -> (w493:string)
      n291 = Format Into String(format string="#%s#" ("初始字符串"), w492) -> (resulting string=w506:string)  [unwired: 2 in, 1 out]
      n292 = Format Into String(format string="#%s#" ("初始字符串"), w496) -> (resulting string=w510:string)  [unwired: 2 in, 1 out]
      n293 = Concatenate Strings("where 参数 ='" ("condition"), w493, "' and 时间 between ", w510, "and" ("字符串"), w506) -> (w498:string)
      n294 = call "SQL查询.vi"("condition"=w498, "table输入"=w494, "database"="database1.mdb") -> ("error out"=w500:errorcluster, "data"=w497:string[][])  [unwired: 7 in]
      n295 = case shown="假" FALSE {
        tunnel: [w520 w523] -> w502
        tunnel: w497 -> [w520 w522]
        tunnel: w500 -> [w519 w521]
        tunnel: [w519 w521] -> w499
        frame False {
        }
        frame True {
          # "数字字符串精度转换保留"
          n296 = Index Array(array=w522, index (col)=3 ("禁用的索引 (列)")) -> (element=w529:string[])  [unwired: 1 in]
          n297 = for {
            tunnel: w529 -> [w532] mode=indexing
            tunnel: [w531] -> w525 mode=indexing
            n298 = Fract/Exp String To Number(string=w532) -> (number=w533:dbl)  [unwired: 3 in, 1 out]
            n299 = Number To Fractional String(number=w533, precision (6)=i16 2 ("精度(6)")) -> (F-format string=w531:string)  [unwired: 2 in]
          }
          n300 = Delete From Array(array=w522, length=1 ("长度"), index (col)=3 ("禁用的索引 (列)")) -> (array with subset deleted=w526:string[][])  [unwired: 1 in, 1 out]
          n301 = Insert Into Array(array=w526, index (col)=3 ("禁用的索引 (列)"), new element=w525) -> (w523:string[][])  [unwired: 1 in]
        }
      }
      n302 = case shown="\"CODCr\", \"总氮\", \"总磷\"" w494 {
        tunnel: w494 -> [_ w518]
        tunnel: w498 -> [_ w517]
        tunnel: w497 -> [_ w516]
        frame Default {
        }
        frame "CODCr", "总氮", "总磷" {
          n303 = global write "全局 实时数据参数.vi" "参数"(w518) -> ()
          n304 = global write "全局 实时数据参数.vi" "连接的字符串"(w517) -> ()
          n305 = global write "全局 实时数据参数.vi" "data"(w516) -> ()
        }
      }
    }
    frame "提取平行样" {
      w537 = "平行样测试" ("字符串")
      # "上传本地时间点的实时数据"
      n306 = global read "全局 数据发送重叠.vi" "掉线指示灯"() -> (w538:bool)
      n307 = case shown="假" w538 {
        tunnel: [w554 w558] -> w539
        frame False {
          n308 = global read "全局 数据发送重叠.vi" "数据发送重叠"() -> (w555:bool)
          n309 = case shown="假" w555 {
            tunnel: [w556 w557] -> w554
            frame False {
              n310 = global read "起始时间.vi" "起始时间"() -> (w556:string)
            }
            frame True {
              n311 = global read "全局 数据发送重叠.vi" "数据发送重叠开始时间戳"() -> (w557:string)
            }
          }
        }
        frame True {
          n312 = global read "全局 数据发送重叠.vi" "TCP掉线时间节点"() -> (w558:string)
        }
      }
      n313 = global read "起始时间.vi" "结束时间"() -> (w535:string)
      n314 = local read "查询元素输入"() -> (w536:string)
      n315 = Format Into String(format string="#%s#" ("初始字符串"), w535) -> (resulting string=w549:string)  [unwired: 2 in, 1 out]
      n316 = Format Into String(format string="#%s#" ("初始字符串"), w539) -> (resulting string=w553:string)  [unwired: 2 in, 1 out]
      n317 = Concatenate Strings("where 参数 ='" ("condition"), w536, "' and 时间 between ", w553, "and" ("字符串"), w549) -> (w541:string)
      n318 = call "SQL查询.vi"("condition"=w541, "table输入"=w537, "database"="database1.mdb") -> ("error out"=w543:errorcluster, "data"=w540:string[][])  [unwired: 7 in]
      n319 = case shown="假" FALSE {
        tunnel: [w563 w566] -> w545
        tunnel: w540 -> [w563 w565]
        tunnel: w543 -> [w562 w564]
        tunnel: [w562 w564] -> w542
        frame False {
        }
        frame True {
          # "数字字符串精度转换保留"
          n320 = Index Array(array=w565, index (col)=3 ("禁用的索引 (列)")) -> (element=w572:string[])  [unwired: 1 in]
          n321 = for {
            tunnel: w572 -> [w575] mode=indexing
            tunnel: [w574] -> w568 mode=indexing
            n322 = Fract/Exp String To Number(string=w575) -> (number=w576:dbl)  [unwired: 3 in, 1 out]
            n323 = Number To Fractional String(number=w576, precision (6)=i16 2 ("精度(6)")) -> (F-format string=w574:string)  [unwired: 2 in]
          }
          n324 = Delete From Array(array=w565, length=1 ("长度"), index (col)=3 ("禁用的索引 (列)")) -> (array with subset deleted=w569:string[][])  [unwired: 1 in, 1 out]
          n325 = Insert Into Array(array=w569, index (col)=3 ("禁用的索引 (列)"), new element=w568) -> (w566:string[][])  [unwired: 1 in]
        }
      }
      n326 = case shown="\"CODCr\", \"总氮\", \"总磷\"" w537 {
        tunnel: w537 -> [_ w561]
        tunnel: w541 -> [_ w560]
        tunnel: w540 -> [_ w559]
        frame Default {
        }
        frame "CODCr", "总氮", "总磷" {
          n327 = global write "全局 实时数据参数.vi" "参数"(w561) -> ()
          n328 = global write "全局 实时数据参数.vi" "连接的字符串"(w560) -> ()
          n329 = global write "全局 实时数据参数.vi" "data"(w559) -> ()
        }
      }
    }
    frame "提取集成干预" {
      w580 = "集成干预测试" ("字符串")
      # "上传本地时间点的实时数据"
      n330 = global read "全局 数据发送重叠.vi" "掉线指示灯"() -> (w581:bool)
      n331 = case shown="假" w581 {
        tunnel: [w597 w601] -> w582
        frame False {
          n332 = global read "全局 数据发送重叠.vi" "数据发送重叠"() -> (w598:bool)
          n333 = case shown="假" w598 {
            tunnel: [w599 w600] -> w597
            frame False {
              n334 = global read "起始时间.vi" "起始时间"() -> (w599:string)
            }
            frame True {
              n335 = global read "全局 数据发送重叠.vi" "数据发送重叠开始时间戳"() -> (w600:string)
            }
          }
        }
        frame True {
          n336 = global read "全局 数据发送重叠.vi" "TCP掉线时间节点"() -> (w601:string)
        }
      }
      n337 = global read "起始时间.vi" "结束时间"() -> (w578:string)
      n338 = local read "查询元素输入"() -> (w579:string)
      n339 = Format Into String(format string="#%s#" ("初始字符串"), w578) -> (resulting string=w592:string)  [unwired: 2 in, 1 out]
      n340 = Format Into String(format string="#%s#" ("初始字符串"), w582) -> (resulting string=w596:string)  [unwired: 2 in, 1 out]
      n341 = Concatenate Strings("where 参数 ='" ("condition"), w579, "' and 时间 between ", w596, "and" ("字符串"), w592) -> (w584:string)
      n342 = call "SQL查询.vi"("condition"=w584, "table输入"=w580, "database"="database1.mdb") -> ("error out"=w586:errorcluster, "data"=w583:string[][])  [unwired: 7 in]
      n343 = case shown="假" FALSE {
        tunnel: [w606 w609] -> w588
        tunnel: w583 -> [w606 w608]
        tunnel: w586 -> [w605 w607]
        tunnel: [w605 w607] -> w585
        frame False {
        }
        frame True {
          # "数字字符串精度转换保留"
          n344 = Index Array(array=w608, index (col)=3 ("禁用的索引 (列)")) -> (element=w615:string[])  [unwired: 1 in]
          n345 = for {
            tunnel: w615 -> [w618] mode=indexing
            tunnel: [w617] -> w611 mode=indexing
            n346 = Fract/Exp String To Number(string=w618) -> (number=w619:dbl)  [unwired: 3 in, 1 out]
            n347 = Number To Fractional String(number=w619, precision (6)=i16 2 ("精度(6)")) -> (F-format string=w617:string)  [unwired: 2 in]
          }
          n348 = Delete From Array(array=w608, length=1 ("长度"), index (col)=3 ("禁用的索引 (列)")) -> (array with subset deleted=w612:string[][])  [unwired: 1 in, 1 out]
          n349 = Insert Into Array(array=w612, index (col)=3 ("禁用的索引 (列)"), new element=w611) -> (w609:string[][])  [unwired: 1 in]
        }
      }
      n350 = case shown="\"CODCr\", \"总氮\", \"总磷\"" w580 {
        tunnel: w580 -> [_ w604]
        tunnel: w584 -> [_ w603]
        tunnel: w583 -> [_ w602]
        frame Default {
        }
        frame "CODCr", "总氮", "总磷" {
          n351 = global write "全局 实时数据参数.vi" "参数"(w604) -> ()
          n352 = global write "全局 实时数据参数.vi" "连接的字符串"(w603) -> ()
          n353 = global write "全局 实时数据参数.vi" "data"(w602) -> ()
        }
      }
    }
    frame "提取实时数据" {
      # "上传给定时间段之间的实时数据"
      n354 = global read "起始时间.vi" "起始时间"() -> (w630:string)
      n355 = global read "起始时间.vi" "结束时间"() -> (w629:string)
      n356 = local read "查询元素输入"() -> (w634:string)
      n357 = global read "全局 实时数据参数.vi" "实时数据参数"() -> (w622:string)
      n358 = Format Into String(format string="#%s#" ("初始字符串"), w630) -> (resulting string=w638:string)  [unwired: 2 in, 1 out]
      n359 = Format Into String(format string="#%s#" ("初始字符串"), w629) -> (resulting string=w631:string)  [unwired: 2 in, 1 out]
      n360 = Concatenate Strings("where 测量模式 ='" ("condition"), w622, "' and 时间 between ", w638, "and" ("字符串"), w631) -> (w636:string)
      n361 = call "SQL查询.vi"("condition"=w636, "table输入"=w634, "database"="database1.mdb") -> ("error out"=w626:errorcluster, "data"=w628:string[][])  [unwired: 7 in]
      n362 = case shown="假" FALSE {
        tunnel: w628 -> [w640 w648]
        tunnel: [w640 w642] -> w627
        tunnel: w626 -> [w639 w641]
        tunnel: [w639 w641] -> w625
        frame False {
        }
        frame True {
          # "数字字符串精度转换保留"
          n363 = Index Array(array=w648, index (col)=3 ("禁用的索引 (列)")) -> (element=w649:string[])  [unwired: 1 in]
          n364 = for {
            tunnel: w649 -> [w652] mode=indexing
            tunnel: [w651] -> w644 mode=indexing
            n365 = Fract/Exp String To Number(string=w652) -> (number=w653:dbl)  [unwired: 3 in, 1 out]
            n366 = Number To Fractional String(number=w653, precision (6)=i16 2 ("精度(6)")) -> (F-format string=w651:string)  [unwired: 2 in]
          }
          n367 = Delete From Array(array=w648, length=1 ("长度"), index (col)=3 ("禁用的索引 (列)")) -> (array with subset deleted=w645:string[][])  [unwired: 1 in, 1 out]
          n368 = Insert Into Array(array=w645, index (col)=3 ("禁用的索引 (列)"), new element=w644) -> (w642:string[][])  [unwired: 1 in]
        }
      }
    }
  }
  "待发送数据" <- w1
  n369 = local write "获取有效数据"(string[][] []) -> ()
  n370 = call <vilib>:"Clear Errors.vi"("error in (no error)"=w6) -> ("error out"=→"error out":errorcluster)  [unwired: 5 in, 1 out]
  n371 = Index Array(array=w1, index (row)=0 ("索引 (行)")) -> (element=→"待发送第一条数据":string[])  [unwired: 1 in]
